vi "Tosca-Quit AI TCP Server.vi"() -> (15 "error out":errorcluster)   [LabVIEW 2020]
uses:
  epl-vi-lib/TCP VIs/TCP Params.ctl
  Sub VIs/Tosca-Globals.vi
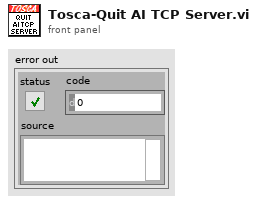
[diagram p1: front panel]
types:
  T1 = typedef "TCP Params.ctl" = cluster{"IP Address":string, "Port":i32}
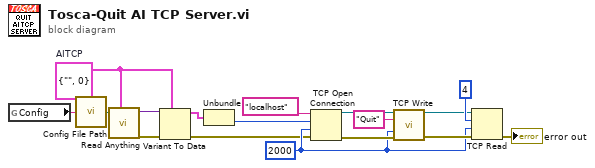
[diagram p0: block diagram]
diagram:
  w6 = T1 {"IP Address"="", "Port"=0}  # AITCP
  w11 = 2000 ("timeout ms (60000)")
  n1 = global read "Tosca-Globals.vi" "Config"() -> (w1:string)
  n2 = call "Config File Path.vi"("AppName"=w1) -> ("Default config file name"=w5:path)
  n3 = call "Read Anything.vi"("Type of Anything"=w6, "Path (dialog)"=w5) -> ("Error Out"=w2:errorcluster, "Anything"=w7:variant)  [unwired: 7 in, 1 out]
  n4 = Variant To Data(error in=w2, type=w6, Variant=w7) -> (data=w8:T1, error out=w3:errorcluster)
  n5 = Unbundle(w8) -> ("Port"=w4:i32)  [unwired: 1 out]
  n6 = TCP Open Connection(address="localhost", remote port or service name=w4, timeout ms (60000)=w11, error in (no error)=w3) -> (connection ID=w17:refnum<k5>, error out=w16:errorcluster)  [unwired: 1 in]
  n7 = call "TCP Write.vi"("connection ID"=w17, "data string"="Quit", "timeout (ms)"=w11, "error in (no error)"=w16) -> ("connection ID out"=w13:refnum<k5>, "error out"=w12:errorcluster)  [unwired: 9 in, 1 out]
  n8 = TCP Read(connection ID=w13, bytes to read=4, error in (no error)=w12, 9:w11) -> (error out=→"error out":errorcluster)  [unwired: 1 in, 2 out]
